vi "Matches.vi"(8 "error in (no error)":errorcluster, 10 "Actual":variant, 11 "Is Less Than in":refnum<class "Is Less Than.lvclass">) -> (0 "error out":errorcluster, 2 "Result":bool, 3 "Is Less Than out":refnum<class "Is Less Than.lvclass">)   [LabVIEW 2017, in "Transparent Assertions.lvlib" / "Is Less Than.lvclass"]
doc: "Evaluates the constraint for <B>Actual</B>. Returns true if the constraint is met."
uses:
  Is Less Than.lvclass
  Is Less Than.lvclass/Is Less Than.ctl
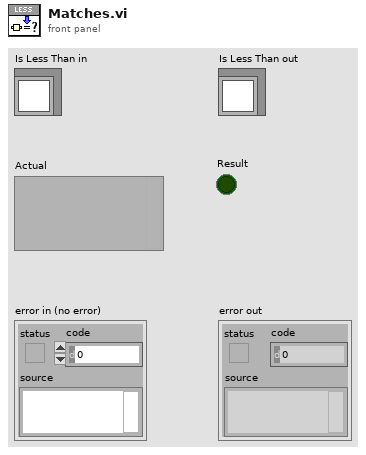
[diagram p1: front panel]
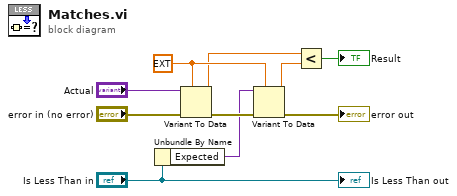
[diagram p0: block diagram]
diagram:
  w3 = ext 0.0
  n1 = Unbundle By Name("Is Less Than in") -> ("Expected"=w5:variant)
  n2 = Variant To Data(error in="error in (no error)", type=w3, Variant="Actual") -> (data=w2:ext, error out=w7:errorcluster)
  n3 = Variant To Data(error in=w7, type=w3, Variant=w5) -> (data=w1:ext, error out=→"error out":errorcluster)
  n4 = Less?(x=w2, y=w1) -> (x < y?=→"Result":bool)
  "Is Less Than out" <- "Is Less Than in"
